vi "RTD_init.vi"(7 "type":T1=enum."COMET Tx5xx (ethernet)" caption="Type", 8 "error in":errorcluster, 11 "VISA in":refnum<visa-resource-name>) -> (0 "error out":errorcluster, 2 "ID":string, 3 "VISA out":refnum<visa-resource-name>)   [LabVIEW 2020]
uses:
  thermo_types.ctl
  drivers/HP34401A/Agilent 34401.lvlib
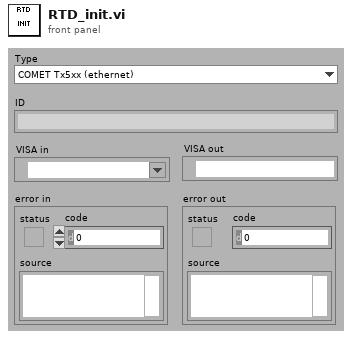
[diagram p1: front panel]
types:
  T1 = typedef "thermo_types.ctl" = enum16{"Disabled", "Simulated", "COMET Tx5xx (ethernet)", "Keithley 2002 (GPIB) + RTD", "Agilent 344xx (GPIB) + RTD"}
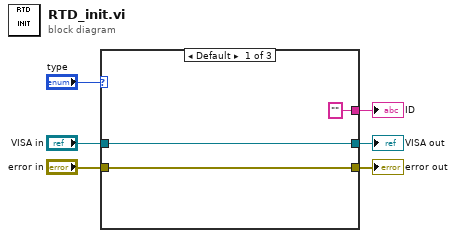
[diagram p0: block diagram]
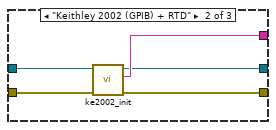
[diagram p2: hidden frame]
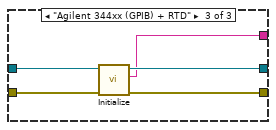
[diagram p3: hidden frame]
diagram:
  n1 = case shown="Default" "type" {
    tunnel: "error in" -> [w9 w14 w19]
    tunnel: [w9 w11 w17] -> w4
    tunnel: [w8 w10 w16] -> w3
    tunnel: "VISA in" -> [w8 w13 w18]
    tunnel: ["" ("id") w12 w15] -> w2
    frame Default {
    }
    frame "Keithley 2002 (GPIB) + RTD" {
      n2 = call "ke2002_init.vi"("error in"=w14, "VISA in"=w13) -> ("error out"=w11:errorcluster, "ID"=w12:string, "VISA out"=w10:refnum<visa-resource-name>)  [unwired: 7 in]
    }
    frame "Agilent 344xx (GPIB) + RTD" {
      n3 = call "Initialize.vi"("error in (no error)"=w19, "VISA resource name"=w18) -> ("error out"=w17:errorcluster, "id"=w15:string, "VISA resource name out"=w16:refnum<visa-resource-name>)  [unwired: 7 in]
    }
  }
  "error out" <- w4
  "VISA out" <- w3
  "ID" <- w2
